vi "Delete Test File.vi"(10 "name or relative path":path, 11 "VI in":refnum<vi>) -> (0 "error out":errorcluster, 2 "deleted path":path)   [LabVIEW 2020, in "Test Open Xml.lvclass"]
uses:
  Test Open Xml.lvclass
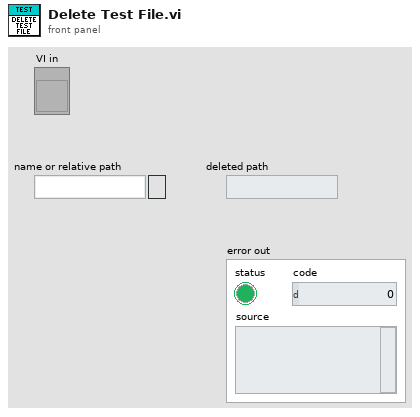
[diagram p1: front panel]
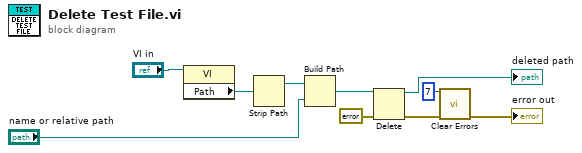
[diagram p0: block diagram]
diagram:
  n1 = property class="VI"(reference="VI in") -> ("Path"=w2:path)  [unwired: 1 in, 2 out]
  n2 = Strip Path(path=w2) -> (stripped path=w3:path)  [unwired: 1 out]
  n3 = Build Path(base path=w3, name or relative path="name or relative path") -> (appended path=w10:path)
  n4 = Delete(path (use dialog)=w10, error in=errorcluster {"status"=FALSE, "code"=0, "source"=""}) -> (deleted path=→"deleted path":path, error out=w6:errorcluster)  [unwired: 3 in, 1 out]
  n5 = call <vilib>:"Clear Errors.vi"("error in (no error)"=w6, "specific error code to clear (0: all)"=7) -> ("error out"=→"error out":errorcluster)  [unwired: 4 in, 1 out]
